vi "shutdown.vi"   [LabVIEW 2017, in "HapticSTM.lvlib"]
doc: "extern \"C\" __declspec(dllexport) void shutdown();"
uses:
  HapticSTM.lvlib
  <userlib>/HapticSTM/HapticSTM.dll
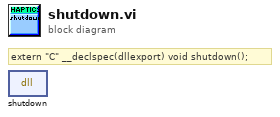
[diagram p0: block diagram]
diagram:
  # "extern \"C\" __declspec(dllexport) void shutdown();"
  n1 = dll-call lib="C:/Program Files/National Instruments/LabVIEW 2017/user.lib/HapticSTM/HapticSTM.*" fn="shutdown"() -> ()  [unwired: 4 in, 2 out]
